vi "ConfigureChannelsForMCSA.vi"(6 "Supported Metrics":string[](array[string]), 8 "error in (no error)":errorcluster, 9 "metric cache":variant, 11 "device":T6) -> (0 "error out":errorcluster, 2 "Motor Info Out":T1, 3 "channels":T2[](array[typedef]))   [LabVIEW 2017, in "McsaAnalysisFunctions.lvlib"]
uses:
  <vilib>/addons/InsightCM/Utilities/Analysis/MCSA/McsaAnalysisFunctions.lvlib
  <vilib>/addons/InsightCM/MessageBus/Base/controls/R2_DeviceModel.ctl
  <vilib>/addons/InsightCM/MessageBus/Base/controls/R2_Device.ctl
  <vilib>/addons/InsightCM/MessageBus/Base/controls/KeyValuePair.ctl
  <vilib>/addons/InsightCM/MessageBus/Base/controls/DeviceState.ctl
  <vilib>/addons/InsightCM/MessageBus/Base/controls/R2_DataGroup.ctl
  <vilib>/addons/InsightCM/MessageBus/Base/controls/OperatingState.ctl
  <vilib>/addons/InsightCM/MessageBus/Base/controls/Trigger.ctl
  <vilib>/addons/InsightCM/MessageBus/Base/controls/Condition.ctl
  <vilib>/addons/InsightCM/MessageBus/Base/controls/BurstModeTrigger.ctl
  <vilib>/addons/InsightCM/MessageBus/Base/controls/R2_Channel.ctl
  <vilib>/addons/InsightCM/MessageBus/Base/controls/Metric.ctl
  <vilib>/addons/InsightCM/MessageBus/Base/controls/Tag.ctl
  <vilib>/addons/InsightCM/Utilities/Analysis/MCSA/controls/McsaChannel.ctl
  <vilib>/addons/InsightCM/Utilities/Analysis/Shared/controls/Feature.ctl
  <vilib>/addons/InsightCM/Utilities/Analysis/Shared/controls/AmplitudeScale.ctl
  <vilib>/addons/InsightCM/Utilities/Analysis/MCSA/controls/McsaMotor.ctl
  <vilib>/addons/InsightCM/Utilities/PropertyHelpers/PropertyHelpers.lvlib
  <vilib>/addons/InsightCM/Utilities/Analysis/Shared/AnalysisHelper.lvlib
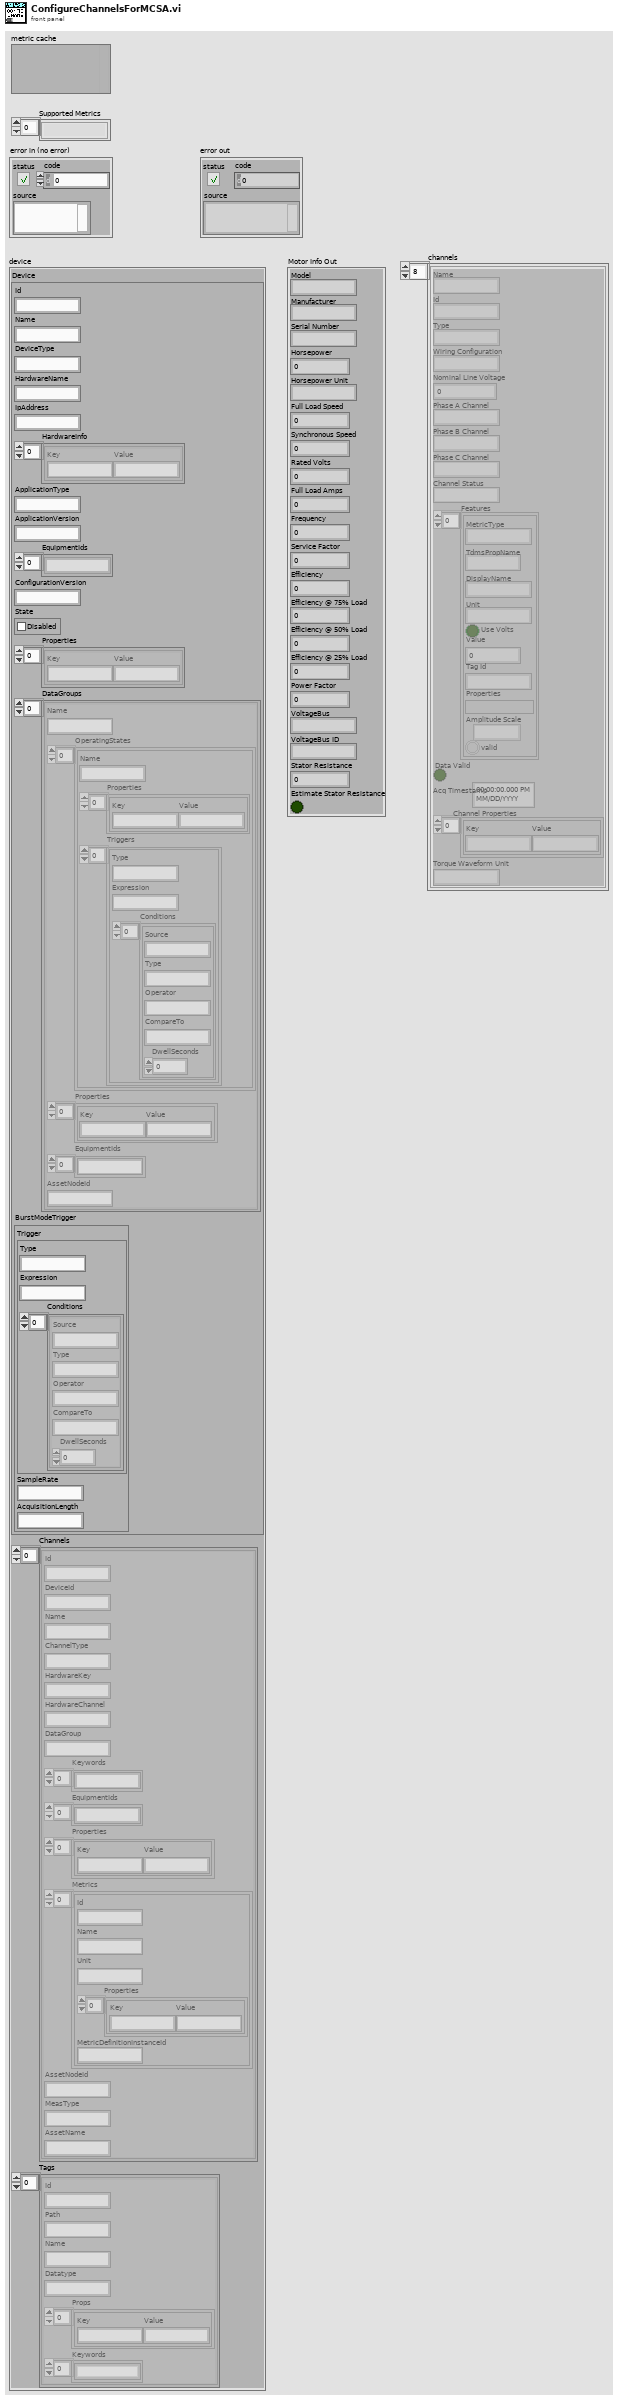
[diagram p1: front panel]
types:
  T1 = typedef "McsaAnalysisFunctions.lvlib/McsaMotor.ctl" = cluster{"Model":string, "Manufacturer":string, "Serial Number":string, "Horsepower":dbl, "Horsepower Unit":string, "Full Load Speed":dbl, "Synchronous Speed":dbl, "Rated Volts":dbl, "Full Load Amps":dbl, "Frequency":dbl, "Service Factor":dbl, "Efficiency":dbl, "Efficiency @ 75% Load":dbl, "Efficiency @ 50% Load":dbl, "Efficiency @ 25% Load":dbl, "Power Factor":dbl, "VoltageBus":string, "VoltageBus ID":string, "Stator Resistance":dbl, "Estimate Stator Resistance":bool}
  T2 = typedef "McsaAnalysisFunctions.lvlib/McsaChannel.ctl" = cluster{"Name":string, "Id":string, "Type":string, "Wiring Configuration":string, "Nominal Line Voltage":dbl, "Phase A Channel":string, "Phase B Channel":string, "Phase C Channel":string, "Channel Status":string, "Features":T3[], "Data Valid":bool, "Acq Timestamp":timestamp, "Channel Properties":T5[], "Torque Waveform Unit":string}
  T3 = typedef "AnalysisHelper.lvlib/Feature.ctl" = cluster{"MetricType":string, "TdmsPropName":string, "DisplayName":string, "Unit":string, "Use Volts":bool, "Value":dbl, "Tag Id":string, "Properties":variant, "Amplitude Scale":T4, "valid":bool}
  T4 = typedef "AnalysisHelper.lvlib/AmplitudeScale.ctl" = enum16{"rms", "peak", "pk-pk"}
  T5 = typedef "KeyValuePair.ctl" = cluster{"Key":string, "Value":string}
  T6 = typedef "R2_DeviceModel.ctl" = cluster{"Device":T7, "Channels":T14[], "Tags":T16[]}
  T7 = typedef "R2_Device.ctl" = cluster{"Id":string, "Name":string, "DeviceType":string, "HardwareName":string, "IpAddress":string, "HardwareInfo":T5[], "ApplicationType":string, "ApplicationVersion":string, "EquipmentIds":string[], "ConfigurationVersion":string, "State":T8, "Properties":T5[], "DataGroups":T9[], "BurstModeTrigger":T13}
  T8 = typedef "DeviceState.ctl" = cluster{"Disabled":bool}
  T9 = typedef "R2_DataGroup.ctl" = cluster{"Name":string, "OperatingStates":T10[], "Properties":T5[], "EquipmentIds":string[], "AssetNodeId":string}
  T10 = typedef "OperatingState.ctl" = cluster{"Name":string, "Properties":T5[], "Triggers":T11[]}
  T11 = typedef "Trigger.ctl" = cluster{"Type":string, "Expression":string, "Conditions":T12[]}
  T12 = typedef "Condition.ctl" = cluster{"Source":string, "Type":string, "Operator":string, "CompareTo":string, "DwellSeconds":dbl}
  T13 = typedef "BurstModeTrigger.ctl" = cluster{"Trigger":T11, "SampleRate":string, "AcquisitionLength":string}
  T14 = typedef "R2_Channel.ctl" = cluster{"Id":string, "DeviceId":string, "Name":string, "ChannelType":string, "HardwareKey":string, "HardwareChannel":string, "DataGroup":string, "Keywords":string[], "EquipmentIds":string[], "Properties":T5[], "Metrics":T15[], "AssetNodeId":string, "MeasType":string, "AssetName":string}
  T15 = typedef "Metric.ctl" = cluster{"Id":string, "Name":string, "Unit":string, "Properties":T5[], "MetricDefinitionInstanceId":string}
  T16 = typedef "Tag.ctl" = cluster{"Id":string, "Path":string, "Name":string, "Datatype":string, "Props":T5[], "Keywords":string[]}
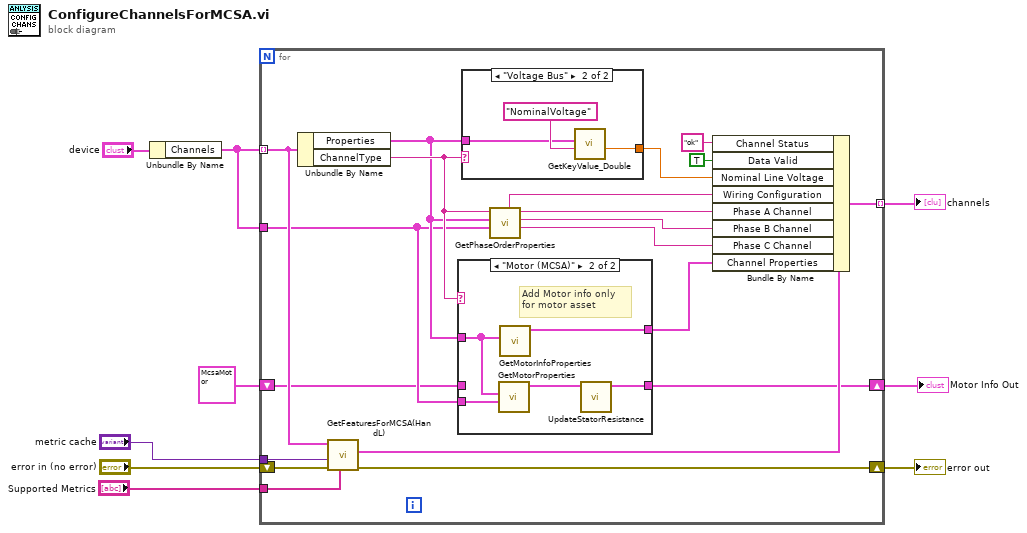
[diagram p0: block diagram]
diagram:
  n1 = Unbundle By Name("device") -> ("Channels"=w5:T14[])
  n2 = for {
    tunnel: [w26] -> w3 mode=indexing
    tunnel: "metric cache" -> [w28]
    tunnel: w5 -> [w27] mode=indexing
    shift-right: [w22] -> w6
    shift-left: "error in (no error)" -> [w29]
    tunnel: w5 -> [w12]
    tunnel: "Supported Metrics" -> [w24]
    shift-right: [w11] -> w1
    shift-left: T1 {"Model"="", "Manufacturer"="", "Serial Number"="", "Horsepower"=0.0, "Horsepower Unit"="", "Full Load Speed"=0.0, "Synchronous Speed"=0.0, "Rated Volts"=0.0, "Full Load Amps"=0.0, "Frequency"=0.0, "Service Factor"=0.0, "Efficiency"=0.0, "Efficiency @ 75% Load"=0.0, "Efficiency @ 50% Load"=0.0, "Efficiency @ 25% Load"=0.0, "Power Factor"=0.0, "VoltageBus"="", "VoltageBus ID"="", "Stator Resistance"=0.0, "Estimate Stator Resistance"=FALSE} ("Motor Info Out") -> [w10]
    n3 = Unbundle By Name(w27) -> ("Properties"=w13:T5[], "ChannelType"=w14:string)
    n4 = call <vilib>:"GetFeaturesForMCSA(HandL).vi"("supported metrics"=w24, "error in (no error)"=w29, "Metric Cache"=w28, "ChannelModel"=w27) -> ("error out"=w22:errorcluster, "channel"=w23:T2)  [unwired: 6 in]
    n5 = case shown="\"Motor (MCSA)\"" w14 {
      tunnel: w13 -> [_ w31]
      tunnel: [_ w35] -> w16
      tunnel: w12 -> [_ w34]
      tunnel: [w30 w32] -> w11
      tunnel: w10 -> [w30 _]
      frame Default {
      }
      frame "Motor (MCSA)" {
        # "Add Motor info only\nfor motor asset"
        n6 = call <vilib>:"GetMotorProperties.vi"("Channels"=w34, "Channel Properties"=w31) -> ("Motor"=w33:T1)  [unwired: 7 in, 2 out]
        n7 = call <vilib>:"GetMotorInfoProperties.vi"("Channel Properties"=w31) -> ("Selected Channel Properties"=w35:T5[])  [unwired: 9 in, 1 out]
        n8 = call <vilib>:"UpdateStatorResistance.vi"("Motor Info In"=w33) -> ("Motor Info Out"=w32:T1)  [unwired: 10 in]
      }
    }
    n9 = case shown="\"Voltage Bus\"" w14 {
      tunnel: w13 -> [_ w37]
      tunnel: [_ w36] -> w25
      frame Default {
      }
      frame "Voltage Bus" {
        n10 = call <vilib>:"GetKeyValue_Double.vi"("key"="NominalVoltage", "key value pairs"=w37) -> ("value"=w36:dbl)  [unwired: 7 in, 2 out]
      }
    }
    n11 = call <vilib>:"GetPhaseOrderProperties.vi"("Channels"=w12, "Channel Properties"=w13, "ChannelType"=w14) -> ("Phase C ChannelName"=w18:string, "Phase B ChannelName"=w19:string, "Phase A ChannelName"=w20:string, "wiring configuraiton"=w21:string)  [unwired: 4 in, 1 out]
    n12 = Bundle By Name(cluster=w23, "Channel Status"="ok", "Data Valid"=TRUE, "Nominal Line Voltage"=w25, "Wiring Configuration"=w21, "Phase A Channel"=w20, "Phase B Channel"=w19, "Phase C Channel"=w18, "Channel Properties"=w16) -> (w26:T2)
  }
  "channels" <- w3
  "error out" <- w6
  "Motor Info Out" <- w1
